vi "Configure RTD [RTD].vi"(8 "error in (no error)":errorcluster, 9 "resistance (0.0 ohms)":dbl format="%^.2e", 10 "alpha (0.0)":dbl format="%^.2e", 11 "CS++DMM in":refnum<class "CS++DMM.lvclass">) -> (0 "error out":errorcluster, 3 "CS++DMM out":refnum<class "CS++DMM.lvclass">)   [LabVIEW 2013, in "CS++DMM.lvlib" / "CS++DMM.lvclass"]
doc: "This VI configures the alpha and resistance parameters for a resistance temperature device.\n\nThis VI affects the behavior of the instrument only when the IviDmm>Temperature Measurements>Transducer Type [TMP] property is set to IVIDMM_VAL_2_WIRE_RTD or IVIDMM_VAL_4_WIRE_RTD.\n\nNote:\n\n(1) This VI is part of the IviDmmResistanceTemperatureDevice [RTD] extension group.\n\n(2) The driver assumes that you are using a Platinum Resistance Temperature Device."
uses:
  CS++DMM.lvclass
  CSPP_Core/Classes/CS++ProcessVariables/ProcessVariable/PV.lvclass
  PV-Enum.ctl
  CSPP_Core/Classes/CS++ProcessVariables/ProcessVariable/PV.lvclass/PV.ctl
  CS++DMM.lvclass/CS++DMM.ctl
  CSPP_Core/Classes/CS++ProcessVariables/PVConnection/PVConnection.lvclass
  CSPP_Core/Classes/CS++ProcessVariables/ProcessVariable/Write Data.vi
  CSPP_Core/Classes/CS++ProcessVariables/ProcessVariable/Write Timestamp.vi
  CSPP_Core/Classes/CS++ProcessVariables/ProcessVariable/Write Quality.vi
  CSPP_Core/Classes/CS++ProcessVariables/ProcessVariable/Write status.vi
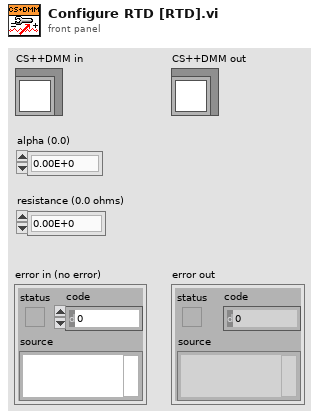
[diagram p1: front panel]
types:
  T1 = typedef "CS++DMM.lvlib/CS++DMM.lvclass/PV-Enum.ctl" = enum16{"AbsoluteResolution", "ACMaxFrequency", "ACMinFrequency", "ActualRange", "Alpha", "ApertureTime", "FixedReferenceJunction", "FrequencyVoltageRange", "PowerLineFrequency", "Range", "Reading", "Resistance", "SampleInterval", "TriggerDelay", "ApertureTimeUnit", "AutoZeroMode", "MeasCompleteDestination", "MeasurementFunction", "ReferenceJunctionType", "SampleCount", "SampleTrigger", "ThermocoupleType", "TranducerType", "TriggerCount", "TriggerSlope", "TriggerSource", "MPReading", "IsOverRange"}
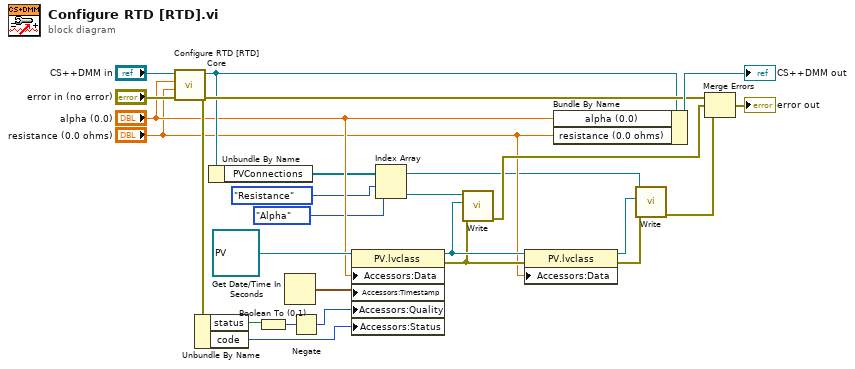
[diagram p0: block diagram]
diagram:
  n1 = call-dynamic "Configure RTD [RTD] Core.vi"("error in (no error)"="error in (no error)", "resistance (0.0 ohms)"="resistance (0.0 ohms)", "alpha (0.0)"="alpha (0.0)", "CS++DMM in"="CS++DMM in") -> ("error out"=w16:errorcluster, "CS++DMM out"=w15:refnum<class "CS++DMM.lvclass">)  [unwired: 6 in]
  n2 = Unbundle By Name(w16) -> ("status"=w21:bool, "code"=w18:i32)
  n3 = Unbundle By Name(w15) -> ("PVConnections"=w5:refnum<class "PVConnection.lvclass">[])
  n4 = Boolean To (0,1)(Boolean=w21) -> (0, 1=w20:i16)
  n5 = Get Date/Time In Seconds() -> (seconds since 1Jan1904=w17:timestamp)
  n6 = Negate(x=w20) -> (-x=w19:i16)
  n7 = property class="PV.lvclass"(reference=refnum<class "PV.lvclass"> refnum ("CS++ProcessVariables.lvlib:PV.lvclass"), "Accessors:Data"="alpha (0.0)", "Accessors:Timestamp"=w17, "Accessors:Quality"=w19, "Accessors:Status"=w18) -> (reference out=w8:refnum<class "PV.lvclass">, error out=w7:errorcluster)  [unwired: 1 in]
  n8 = Index Array(array=w5, index #1=PV-Enum."Resistance" ("PV-Enum"), index #2=PV-Enum."Alpha" ("PV-Enum")) -> (element #1=w4:refnum<class "PVConnection.lvclass">, element #2=w2:refnum<class "PVConnection.lvclass">)
  n9 = call-dynamic "Write.vi"("error in (no error)"=w7, "PV"=w8, "PVConnection in"=w2) -> ("error out"=w10:errorcluster)  [unwired: 7 in, 1 out]
  n10 = property class="PV.lvclass"(reference=w8, error in=w7, "Accessors:Data"="resistance (0.0 ohms)") -> (reference out=w13:refnum<class "PV.lvclass">, error out=w12:errorcluster)
  n11 = Bundle By Name(cluster=w15, "alpha (0.0)"="alpha (0.0)", "resistance (0.0 ohms)"="resistance (0.0 ohms)") -> (→"CS++DMM out":refnum<class "CS++DMM.lvclass">)
  n12 = call-dynamic "Write.vi"("error in (no error)"=w12, "PV"=w13, "PVConnection in"=w4) -> ("error out"=w9:errorcluster)  [unwired: 7 in, 1 out]
  n13 = Merge Errors(w16, w10, w9) -> (→"error out":errorcluster)
